vi "check_instr_type.vi"(5 "Error Generation Mode":T1(ring), 7 "Attribute":T2={"Identifier"="", "Descriptive Name"="", "Data Type"=enum."Integer 32", "Command"="", "Access"=enum."Read/Write", "Range Table"="", "Read Callback"="", "Write Callback"="", "Supported Models"="", "Instrument Options"="", "Index"=0, "OPC Wait"=FALSE, "No Status Check"=FALSE, "Cache Only"=FALSE}, 8 "error in":errorcluster caption="error in (no error)", 11 "VISA resource name":refnum<visa-resource-name>) -> (0 "error out":errorcluster, 2 "Instrument present":bool, 3 "VISA resource name out":refnum<visa-resource-name>)   [LabVIEW 2020, in "Rohde&Schwarz RTx Oscilloscopes.lvlib" / "rsidr_core.lvlib"]
uses:
  rsidr_core.lvlib
  type_Attribute.ctl
  type_Attribute_Data_Type.ctl
  type_ReadWriteAccess.ctl
  type_Error_Codes.ctl
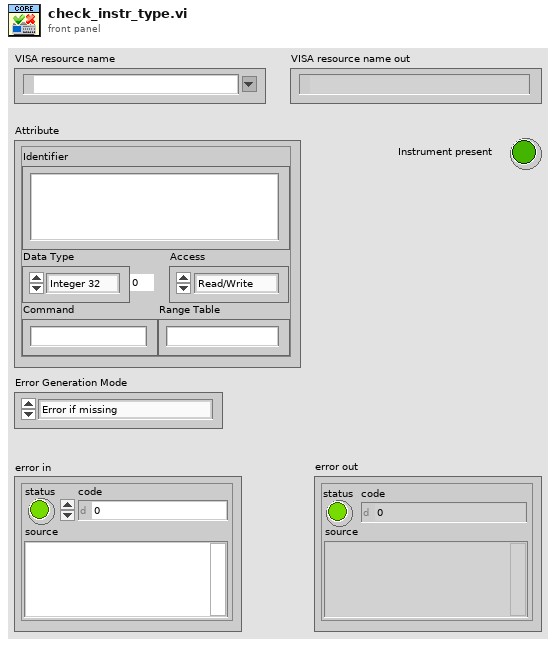
[diagram p1: front panel]
types:
  T1 = enum16{"Error if missing", "Error if present", "No error"}
  T2 = typedef "Rohde&Schwarz RTx Oscilloscopes.lvlib/rsidr_core.lvlib/type_Attribute.ctl" = cluster{"Identifier":string, "Descriptive Name":string, "Data Type":T3, "Command":string, "Access":T4, "Range Table":string, "Read Callback":string, "Write Callback":string, "Supported Models":string, "Instrument Options":string, "Index":i32, "OPC Wait":bool, "No Status Check":bool, "Cache Only":bool}
  T3 = typedef "Rohde&Schwarz RTx Oscilloscopes.lvlib/rsidr_core.lvlib/type_Attribute_Data_Type.ctl" = enum16{"Integer 32", "Double", "String", "Boolean", "None", "Integer 64", "RawString"}
  T4 = typedef "Rohde&Schwarz RTx Oscilloscopes.lvlib/rsidr_core.lvlib/type_ReadWriteAccess.ctl" = enum16{"Read Only", "Write Only", "Read/Write"}
  T5 = typedef "Rohde&Schwarz RTx Oscilloscopes.lvlib/rsidr_core.lvlib/type_Error_Codes.ctl" = enum16{"No_error", "VISA_err_ResourceNotFound", "VISA_err_Timeout", "VISA_warn_MoreDataAvailable", "RS_err_MissingCallback", "RS_err_InvalidAttribute", "RS_err_InvalidValue", "RS_err_UnknownResource", "RS_err_AlreadyInitialized", "RS_err_InstrumentStatus", "RS_err_BadRepCapName", "RS_err_TypesMismatch", "RS_err_ValueNotSupported", "RS_err_InvalidRngTable", "RS_err_IDqueryFail", "RS_err_UnexpResponse", "VISA_warn_ConfigNotLoaded", "RS_err_AttributeNotReadable", "RS_err_AttributeNotWritable", "RS_err_InstrumentType", "RS_err_InstrumentOption", "VISA_err_InvalidSize", "RS_err_ReliabilityIndicator", "VISA_warn_UnknownStatus", "VISA_warn_TermCharRead", "VISA_err_IO_error", "RS_err_FunctionNotSupported", "VISA_warn_QueueEmpty"}
  T6 = typedef "Rohde&Schwarz RTx Oscilloscopes.lvlib/rsidr_core.lvlib/type_Session_Data.ctl" = cluster{"IDN string":string, "Instrument FW":string, "Instr type":string, "Instr type for err. msg.":string, "Installed Options":string[], "Ignore Error Messages":string, "Logging params":variant, "OPC Timeout":i32, "VISA Timeout":i32, "STB Poll VISA Timeout":i32, "Additional Flags":i32, "Wait Before Read":i32, "Wait Before Write":i32, "Option String Flags":i32, "IO Segment Size":i64, "VISA Access Mode":T7, "Interface Type":T8, "OPC Wait Mode":T9, "Bin Float Number  Format":T10, "Bin Integer Number Format":T11, "Simulate":bool, "VXIcapable":bool, "Duplicate Session":bool, "Add LF to Write":bool, "Logging":bool, "Fast Sweep":bool, "Query Instrument Status":bool, "Check Range":bool, "Check Options":bool, "OPC-sync Attr Writes":bool, "OPC-sync Attr Queries":bool}
  T7 = typedef "Rohde&Schwarz RTx Oscilloscopes.lvlib/rsidr_core.lvlib/type_VisaAccessMode.ctl" = u16
  T8 = typedef "Rohde&Schwarz RTx Oscilloscopes.lvlib/rsidr_core.lvlib/type_InterfaceType.ctl" = enum16{"Unknown", "GPIB", "VXI", "GPIB_VXI", "ASRL", "PXI", "TCPIP", "USB", "SOCKET"}
  T9 = typedef "Rohde&Schwarz RTx Oscilloscopes.lvlib/rsidr_core.lvlib/type_OPC_Wait_Mode.ctl" = enum16{"STBpolling", "STBpollingSlow", "STBpollingSuperSlow", "ServiceRequest", "OPCquery"}
  T10 = typedef "Rohde&Schwarz RTx Oscilloscopes.lvlib/rsidr_core.lvlib/type_Binary_Float_Number_Format.ctl" = enum16{"Float_4_Bytes_Swapped", "Float_4_Bytes", "Double_8_Bytes_Swapped", "Double_8_Bytes"}
  T11 = typedef "Rohde&Schwarz RTx Oscilloscopes.lvlib/rsidr_core.lvlib/type_Binary_Integer_Number_Format.ctl" = enum16{"Int32_4_Bytes_Swapped", "Int32_4 Bytes", "Int16_2_Bytes_Swapped", "Int16_2_Bytes"}
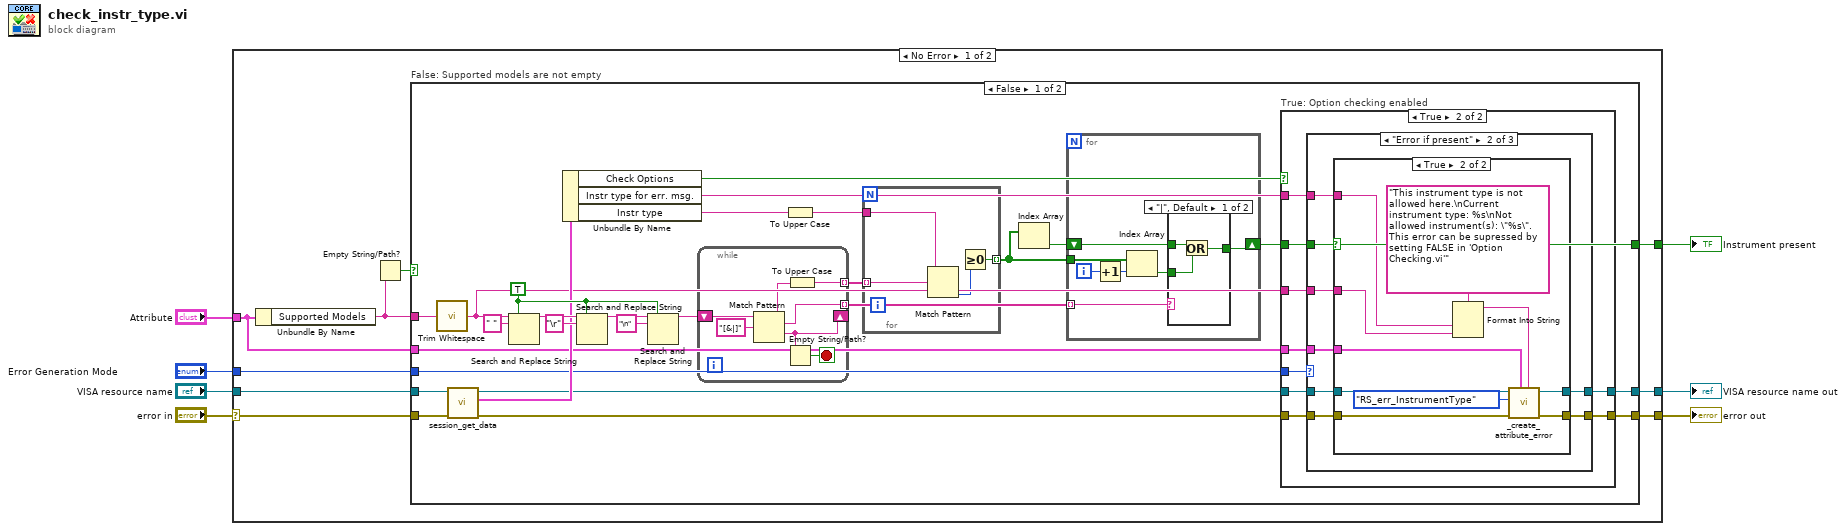
[diagram p0: block diagram]
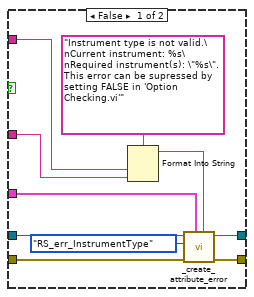
[diagram p4: hidden frame]
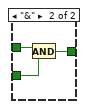
[diagram p7: hidden frame]
diagram:
  n1 = case shown="No Error" "error in" {
    selector: "error in" -> [w10 w123]
    tunnel: [w16 w123] -> w7
    tunnel: "Attribute" -> [w13 _]
    tunnel: "VISA resource name" -> [w11 w124]
    tunnel: [w12 w124] -> w4
    tunnel: [w9 _] -> w2
    tunnel: "Error Generation Mode" -> [w8 _]
    frame No Error {
      n2 = Unbundle By Name(w13) -> ("Supported Models"=w14:string)
      n3 = Empty String/Path?(string/path=w14) -> (empty?=w15:bool)
      n4 = case "False: Supported models are not empty" shown="False" w15 {
        tunnel: w10 -> [w30 w122]
        tunnel: [w23 w122] -> w16
        tunnel: w14 -> [w43 _]
        tunnel: w13 -> [w26 _]
        tunnel: [w20 w121] -> w12
        tunnel: w11 -> [w31 w121]
        tunnel: [w28 _] -> w9
        tunnel: w8 -> [w19 _]
        frame False {
          w33 = TRUE ("replace all? (F)")
          n5 = call "Trim Whitespace.vi"("string"=w43) -> ("trimmed string"=w25:string)  [unwired: 1 in]
          n6 = call "session_get_data.vi"("error in"=w30, "VISA resource name"=w31) -> ("error out"=w24:errorcluster, "Session User Data out"=w29:T6, "VISA resource name out"=w21:refnum<visa-resource-name>)  [unwired: 6 in, 1 out]
          n7 = Search and Replace String(replace all?=w33, input string=w25, search string=" ") -> (result string=w36:string)  [unwired: 5 in, 3 out]
          n8 = Unbundle By Name(w29) -> ("Check Options"=w22:bool, "Instr type for err. msg."=w27:string, "Instr type"=w18:string)
          n9 = Search and Replace String(replace all?=w33, input string=w36, search string="\r") -> (result string=w35:string)  [unwired: 5 in, 3 out]
          n10 = Search and Replace String(replace all?=w33, input string=w35, search string="\n") -> (result string=w34:string)  [unwired: 5 in, 3 out]
          n11 = while {
            shift-right: [w116] -> _
            shift-left: w34 -> [w120]
            tunnel: [w114] -> w32 mode=indexing
            tunnel: [w118] -> w41 mode=indexing
            stop <- w117 stop-if-true
            n12 = Match Pattern(string=w120, regular expression="[&|]") -> (before substring=w115:string, match substring=w118:string, after substring=w116:string)  [unwired: 1 in, 1 out]
            n13 = Empty String/Path?(string/path=w116) -> (empty?=w117:bool)
            n14 = To Upper Case(1:w115) -> (0:w114:string)
          }
          n15 = To Upper Case(1:w18) -> (0:w17:string)
          n16 = for {
            tunnel: w32 -> [w110] mode=indexing
            tunnel: [w113] -> w39 mode=indexing
            tunnel: w17 -> [w111]
            n17 = Match Pattern(string=w111, regular expression=w110) -> (offset past match=w112:i32)  [unwired: 1 in, 3 out]
            n18 = Greater Or Equal To 0?(x=w112) -> (x >= 0?=w113:bool)
          }
          n19 = Index Array(array=w39) -> (element=w40:bool)  [unwired: 1 in]
          n20 = for {
            tunnel: w41 -> [w98] mode=indexing
            tunnel: w39 -> [w102]
            shift-right: [w97] -> w28
            shift-left: w40 -> [w103]
            i -> [w100]
            n21 = Increment(x=w100) -> (x+1=w101:i32)
            n22 = Index Array(array=w102, index=w101) -> (element=w99:bool)
            n23 = case shown="\"|\", Default" w98 {
              tunnel: w103 -> [w105 w109]
              tunnel: [w106 w108] -> w97
              tunnel: w99 -> [w104 w107]
              frame "|", Default {
                n24 = Or(x=w105, y=w104) -> (x .or. y?=w106:bool)
              }
              frame "&" {
                n25 = And(x=w109, y=w107) -> (x .and. y?=w108:bool)
              }
            }
          }
          n26 = case "True: Option checking enabled" shown="True" w22 {
            tunnel: w19 -> [_ w54]
            tunnel: w28 -> [_ w53]
            tunnel: w27 -> [_ w52]
            tunnel: w26 -> [_ w51]
            tunnel: w25 -> [_ w50]
            tunnel: w24 -> [w45 w49]
            tunnel: [w45 w48] -> w23
            tunnel: w21 -> [w44 w47]
            tunnel: [w44 w46] -> w20
            frame False {
            }
            frame True {
              n27 = case shown="\"Error if present\"" w54 {
                tunnel: w53 -> [w62 w82 _]
                tunnel: w52 -> [w60 w80 _]
                tunnel: w51 -> [w61 w81 _]
                tunnel: w50 -> [w59 w79 _]
                tunnel: w49 -> [w58 w78 w96]
                tunnel: [w57 w77 w96] -> w48
                tunnel: w47 -> [w56 w76 w95]
                tunnel: [w55 w75 w95] -> w46
                frame "Error if missing" {
                  n28 = case shown="True" w62 {
                    tunnel: w61 -> [w70 _]
                    tunnel: w60 -> [w69 _]
                    tunnel: w59 -> [w68 _]
                    tunnel: w58 -> [w67 w74]
                    tunnel: [w66 w74] -> w57
                    tunnel: w56 -> [w65 w73]
                    tunnel: [w63 w73] -> w55
                    frame False {
                      n29 = Format Into String(format string="Instrument type is not valid.\nCurrent instrument: %s\nRequired instrument(s): \"%s\". This error can be supressed by setting FALSE in 'Option Checking.vi'" ("string"), w69, w68) -> (resulting string=w72:string)  [unwired: 2 in, 1 out]
                      n30 = call "_create_attribute_error.vi"("Error Elaboration (\"\")"=w72, "Attribute"=w70, "error in"=w67, "Error Enum in"=type_Error_Codes."RS_err_InstrumentType" ("Error Enum in (from err to recompose)"), "VISA resource name"=w65) -> ("error out"=w66:errorcluster, "VISA resource name out"=w63:refnum<visa-resource-name>)  [unwired: 5 in]
                    }
                    frame True {
                    }
                  }
                }
                frame "Error if present" {
                  n31 = case shown="True" w82 {
                    tunnel: w81 -> [_ w92]
                    tunnel: w80 -> [_ w91]
                    tunnel: w79 -> [_ w90]
                    tunnel: w78 -> [w84 w89]
                    tunnel: [w84 w88] -> w77
                    tunnel: w76 -> [w83 w86]
                    tunnel: [w83 w85] -> w75
                    frame False {
                    }
                    frame True {
                      n32 = Format Into String(format string="This instrument type is not allowed here.\nCurrent instrument type: %s\nNot allowed instrument(s): \"%s\". This error can be supressed by setting FALSE in 'Option Checking.vi'" ("string"), w91, w90) -> (resulting string=w94:string)  [unwired: 2 in, 1 out]
                      n33 = call "_create_attribute_error.vi"("Error Elaboration (\"\")"=w94, "Attribute"=w92, "error in"=w89, "Error Enum in"=type_Error_Codes."RS_err_InstrumentType" ("Error Enum in (from err to recompose)"), "VISA resource name"=w86) -> ("error out"=w88:errorcluster, "VISA resource name out"=w85:refnum<visa-resource-name>)  [unwired: 5 in]
                    }
                  }
                }
                frame "No error" {
                }
              }
            }
          }
        }
        frame True {
        }
      }
    }
    frame Error {
    }
  }
  "error out" <- w7
  "VISA resource name out" <- w4
  "Instrument present" <- w2
